vi "Create Queues.vi"(8 "error in":errorcluster) -> (0 "error out":errorcluster, 3 "QRD Out":T1, 5 "Operations Q":refnum<queue>)   [LabVIEW 2025]
uses:
  Controls/Queues-Refs-Data.ctl
  Builds/Queue Wrappers.lvlibp/Q Packet.ctl
  Builds/Queue Wrappers.lvlibp
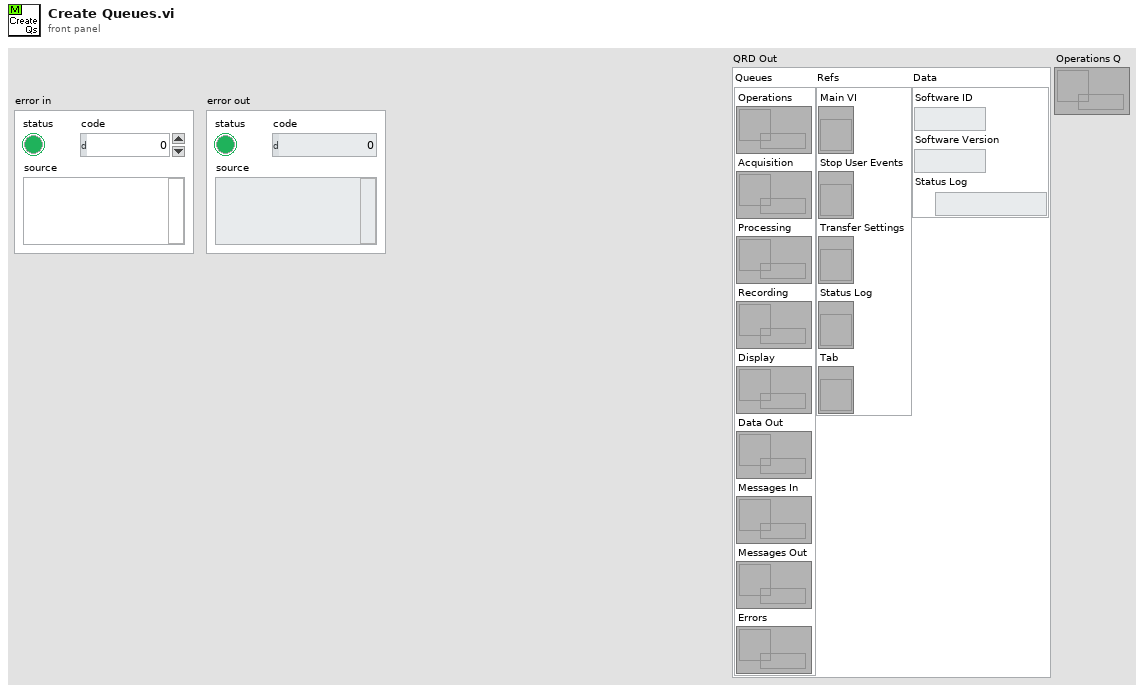
[diagram p1: front panel]
types:
  T1 = typedef "Queues-Refs-Data.ctl" = cluster{"Queues":cluster{"Operations":refnum<queue>, "Acquisition":refnum<queue>, "Processing":refnum<queue>, "Recording":refnum<queue>, "Display":refnum<queue>, "Data Out":refnum<queue>, "Messages In":refnum<queue>, "Messages Out":refnum<queue>, "Errors":refnum<queue>}, "Refs":cluster{"Main VI":refnum<vi>, "Stop User Events":refnum<vi>, "Transfer Settings":refnum<vi>, "Status Log":refnum<vi>, "Tab":refnum<vi>}, "Data":cluster{"Software ID":string, "Software Version":string, "Status Log":path}}
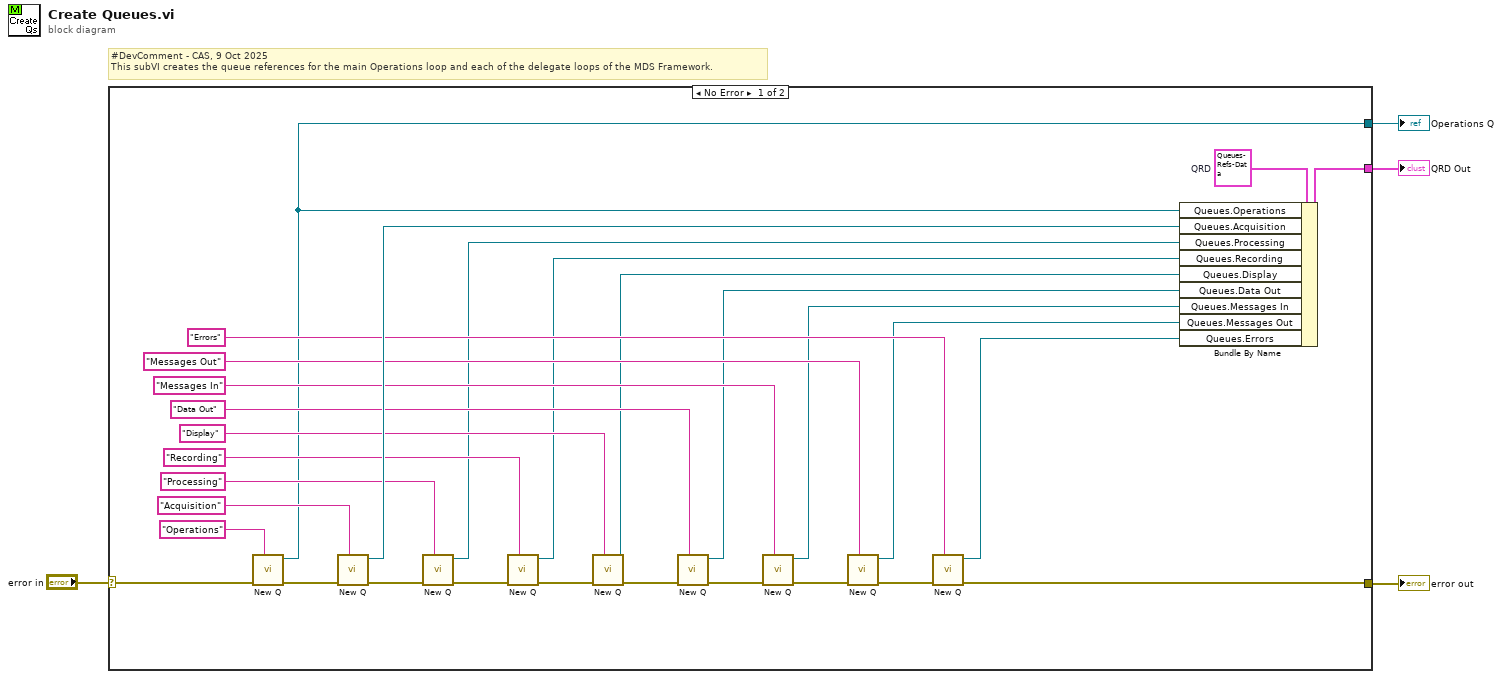
[diagram p0: block diagram]
diagram:
  # "#DevComment - CAS, 9 Oct 2025\nThis subVI creates the queue references for the main Operations loop and each of the delegate loops of the MDS Framework."
  n1 = case shown="No Error" "error in" {
    selector: "error in" -> [w33 w35]
    tunnel: [w14 w35] -> w3
    tunnel: [w34 _] -> w2
    tunnel: [w5 _] -> w1
    frame No Error {
      w6 = T1 {"Queues"={"Operations"=refnum, "Acquisition"=refnum, "Processing"=refnum, "Recording"=refnum, "Display"=refnum, "Data Out"=refnum, "Messages In"=refnum, "Messages Out"=refnum, "Errors"=refnum}, "Refs"={"Main VI"=refnum, "Stop User Events"=refnum, "Transfer Settings"=refnum, "Status Log"=refnum, "Tab"=refnum}, "Data"={"Software ID"="", "Software Version"="", "Status Log"=path ""}}  # QRD
      n2 = call "New Q.vi"("Base Name"="Operations", "error in"=w33) -> ("error out"=w31:errorcluster, "Q Ref Out"=w5:refnum<queue>)  [unwired: 8 in]
      n3 = call "New Q.vi"("Base Name"="Acquisition", "error in"=w31) -> ("error out"=w28:errorcluster, "Q Ref Out"=w29:refnum<queue>)  [unwired: 8 in]
      n4 = call "New Q.vi"("Base Name"="Processing", "error in"=w28) -> ("error out"=w26:errorcluster, "Q Ref Out"=w7:refnum<queue>)  [unwired: 8 in]
      n5 = call "New Q.vi"("Base Name"="Recording", "error in"=w26) -> ("error out"=w24:errorcluster, "Q Ref Out"=w8:refnum<queue>)  [unwired: 8 in]
      n6 = call "New Q.vi"("Base Name"="Display", "error in"=w24) -> ("error out"=w22:errorcluster, "Q Ref Out"=w9:refnum<queue>)  [unwired: 8 in]
      n7 = call "New Q.vi"("Base Name"="Data Out", "error in"=w22) -> ("error out"=w20:errorcluster, "Q Ref Out"=w10:refnum<queue>)  [unwired: 8 in]
      n8 = call "New Q.vi"("Base Name"="Messages In", "error in"=w20) -> ("error out"=w18:errorcluster, "Q Ref Out"=w11:refnum<queue>)  [unwired: 8 in]
      n9 = call "New Q.vi"("Base Name"="Messages Out", "error in"=w18) -> ("error out"=w16:errorcluster, "Q Ref Out"=w12:refnum<queue>)  [unwired: 8 in]
      n10 = call "New Q.vi"("Base Name"="Errors", "error in"=w16) -> ("error out"=w14:errorcluster, "Q Ref Out"=w13:refnum<queue>)  [unwired: 8 in]
      n11 = Bundle By Name(cluster=w6, "Queues.Operations"=w5, "Queues.Acquisition"=w29, "Queues.Processing"=w7, "Queues.Recording"=w8, "Queues.Display"=w9, "Queues.Data Out"=w10, "Queues.Messages In"=w11, "Queues.Messages Out"=w12, "Queues.Errors"=w13) -> (w34:T1)
    }
    frame Error {
    }
  }
  "error out" <- w3
  "QRD Out" <- w2
  "Operations Q" <- w1
